vi "Change Las Parameters.vi"(8 "error in":errorcluster, 10 "lasParam":cluster{"freq":dbl, "duty_cyc":dbl}, 11 "CRDS in":refnum<class "CRDS.lvclass">) -> (0 "error out":errorcluster, 3 "CRDS out":refnum<class "CRDS.lvclass">)   [LabVIEW 2011]
uses:
  CRDS.lvclass
  Program Files/National Instruments/LabVIEW 2011/resource/objmgr/daqmx.rc
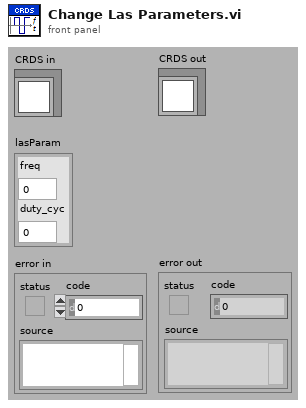
[diagram p1: front panel]
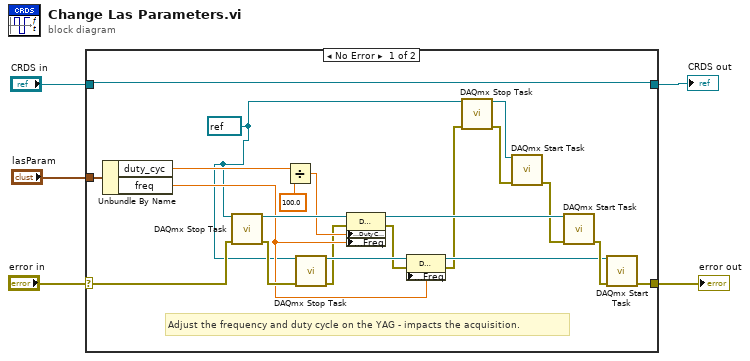
[diagram p0: block diagram]
diagram:
  n1 = case shown="No Error" "error in" {
    selector: "error in" -> [w15 w28]
    tunnel: [w14 w28] -> w4
    tunnel: [w13 w27] -> w2
    tunnel: "CRDS in" -> [w13 w27]
    tunnel: "lasParam" -> [w16 _]
    frame No Error {
      w6 = refnum<k21> refnum ("task/channels in")
      # "Adjust the frequency and duty cycle on the YAG - impacts the acquisition."
      n2 = Unbundle By Name(w16) -> ("duty_cyc"=w19:dbl, "freq"=w24:dbl)
      n3 = call <vilib>:"DAQmx Stop Task.vi"("task/channels in"=w6, "error in"=w15) -> ("task out"=w25:refnum<k21>, "error out"=w26:errorcluster)  [unwired: 12 in]
      n4 = Divide(x=w19, y=100.0) -> (x/y=w17:dbl)
      n5 = call <vilib>:"DAQmx Stop Task.vi"("task/channels in"=w6, "error in"=w26) -> ("task out"=w23:refnum<k21>, "error out"=w12:errorcluster)  [unwired: 12 in]
      n6 = property class="DAQmx Channel"(reference=w25, error in=w12, "CO.Pulse.DutyCyc"=w17, "CO.Pulse.Freq"=w24) -> (reference out=w20:refnum<k21>, error out=w11:errorcluster)
      n7 = property class="DAQmx Channel"(reference=w23, error in=w11, "CO.Pulse.Freq"=w24) -> (reference out=w21:refnum<k21>, error out=w10:errorcluster)
      n8 = call <vilib>:"DAQmx Stop Task.vi"("task/channels in"=w6, "error in"=w10) -> ("task out"=w8:refnum<k21>, "error out"=w9:errorcluster)  [unwired: 12 in]
      n9 = call <vilib>:"DAQmx Start Task.vi"("task/channels in"=w8, "error in"=w9) -> ("error out"=w7:errorcluster)  [unwired: 12 in, 1 out]
      n10 = call <vilib>:"DAQmx Start Task.vi"("task/channels in"=w20, "error in"=w7) -> ("error out"=w22:errorcluster)  [unwired: 12 in, 1 out]
      n11 = call <vilib>:"DAQmx Start Task.vi"("task/channels in"=w21, "error in"=w22) -> ("error out"=w14:errorcluster)  [unwired: 12 in, 1 out]
    }
    frame Error {
    }
  }
  "error out" <- w4
  "CRDS out" <- w2
